vi "Get TCP Messaging Info.vi"(8 "error in (no error)":errorcluster, 11 "Node Config in":refnum<class "Node Config.lvclass">) -> (0 "error out":errorcluster, 2 "TCP Messaging Info":T1, 3 "Node Config out":refnum<class "Node Config.lvclass">)   [LabVIEW 2020, in "VectoConfig.lvlib" / "Node Config.lvclass"]
uses:
  Node Config.lvclass
  TCP Messaging Info.ctl
  Node Config.lvclass/Node Config.ctl
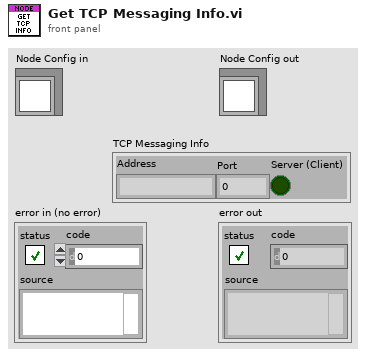
[diagram p1: front panel]
types:
  T1 = typedef "VectoConfig.lvlib/Node Config.lvclass/TCP Messaging Info.ctl" = cluster{"Address":string, "Port":u16, "Server (Client)":bool}
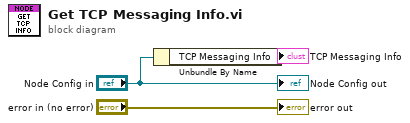
[diagram p0: block diagram]
diagram:
  n1 = Unbundle By Name("Node Config in") -> ("TCP Messaging Info"=→"TCP Messaging Info":T1)
  "error out" <- "error in (no error)"
  "Node Config out" <- "Node Config in"
